vi "Fall2016SemesterPIDController.vi"(0 "Encoder Angle (degrees)":dbl format="%.2f", 1 "Encoder Angle Setpoint (degrees)":dbl format="%.2f", 2 "PID gains":T1={"proportional gain (Kc)"=0.04, "integral time (Ti, min)"=0.0, "derivative time (Td, min)"=0.004} {"derivative time (Td, min)" min=-0.1 max=0.1 step=1e-05 format="%.5f"; "integral time (Ti, min)" min=-10.0 max=10.0 step=1e-05 format="%.5f"; "proportional gain (Kc)" format="%.3f"}, 3 "Spin Frac Min/Max":cluster{"output high":dbl, "output low":dbl}={"output high"=0.5, "output low"=-0.5}, 4 "Old Error":dbl) -> (5 "New Error":dbl, 7 "SpinFraction":dbl)   [LabVIEW 2015]
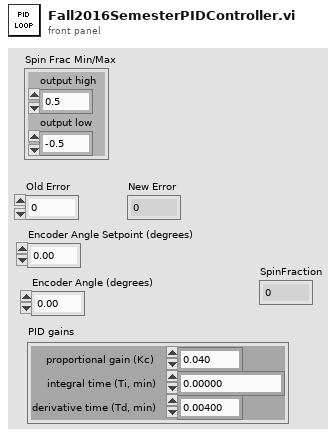
[diagram p1: front panel]
types:
  T1 = cluster{"proportional gain (Kc)":dbl, "integral time (Ti, min)":dbl, "derivative time (Td, min)":dbl}
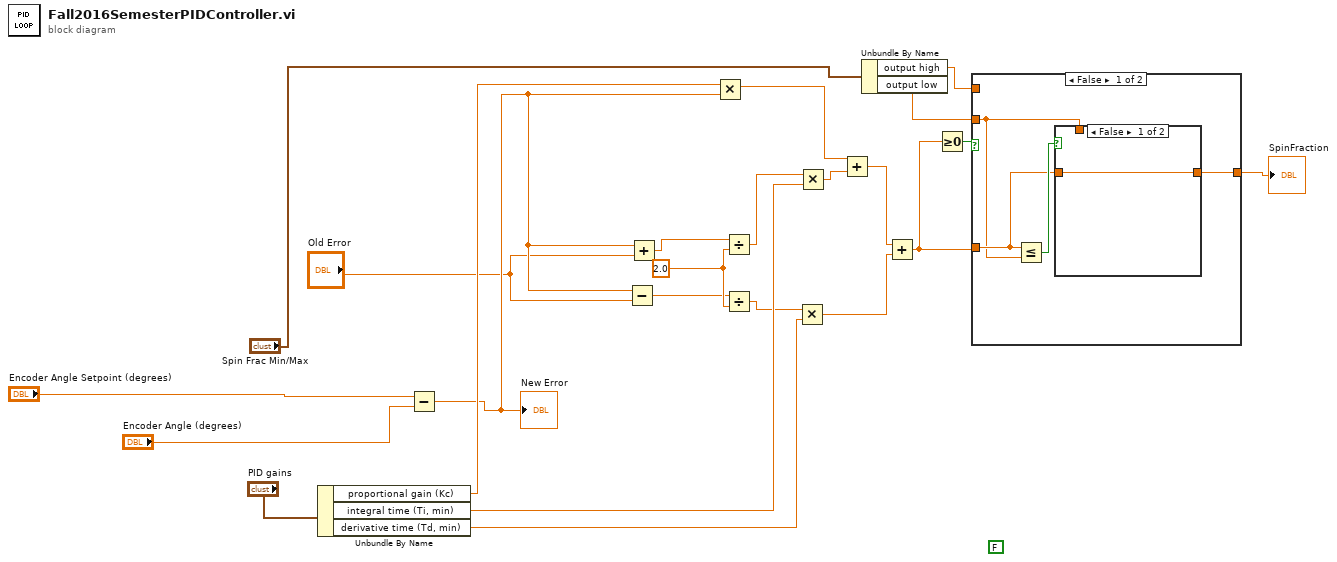
[diagram p0: block diagram]
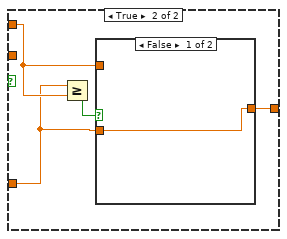
[diagram p3: hidden frame]
diagram:
  (unwired) FALSE
  w15 = 2.0 ("y")
  n1 = Unbundle By Name("PID gains") -> ("proportional gain (Kc)"=w20:dbl, "integral time (Ti, min)"=w18:dbl, "derivative time (Td, min)"=w17:dbl)
  n2 = Subtract(x="Encoder Angle Setpoint (degrees)", y="Encoder Angle (degrees)") -> (x-y=w19:dbl)
  "New Error" <- w19
  n3 = Subtract(x=w19, y="Old Error") -> (x-y=w14:dbl)
  n4 = Add(x=w19, y="Old Error") -> (x+y=w13:dbl)
  n5 = Multiply(x=w20, y=w19) -> (x*y=w10:dbl)
  n6 = Divide(x=w13, y=w15) -> (x/y=w11:dbl)
  n7 = Divide(x=w14, y=w15) -> (x/y=w12:dbl)
  n8 = Multiply(x=w12, y=w17) -> (x*y=w7:dbl)
  n9 = Multiply(x=w11, y=w18) -> (x*y=w9:dbl)
  n10 = Add(x=w10, y=w9) -> (x+y=w8:dbl)
  n11 = Unbundle By Name("Spin Frac Min/Max") -> ("output high"=w5:dbl, "output low"=w3:dbl)
  n12 = Add(x=w8, y=w7) -> (x+y=w2:dbl)
  n13 = Greater Or Equal To 0?(x=w2) -> (x >= 0?=w6:bool)
  n14 = case shown="False" w6 {
    tunnel: w5 -> [_ w31]
    tunnel: w2 -> [w25 w30]
    tunnel: [w26 w32] -> w4
    tunnel: w3 -> [w24 _]
    frame False {
      n15 = Less Or Equal?(x=w25, y=w24) -> (x <= y?=w27:bool)
      n16 = case shown="False" w27 {
        tunnel: [w28 w29] -> w26
        tunnel: w25 -> [w28 _]
        tunnel: w24 -> [_ w29]
        frame False {
        }
        frame True {
        }
      }
    }
    frame True {
      n17 = Greater Or Equal?(x=w30, y=w31) -> (x >= y?=w33:bool)
      n18 = case shown="False" w33 {
        tunnel: [w34 w35] -> w32
        tunnel: w30 -> [w34 _]
        tunnel: w31 -> [_ w35]
        frame False {
        }
        frame True {
        }
      }
    }
  }
  "SpinFraction" <- w4
